vi "z motion pattern_v1.vi"(9 "traj array size":i32, 10 "no of lobes":i8, 11 "Window Array":dbl[](array[numeric])) -> (2 "(cos(n_flr*s/4).^2).*w":dbl[](array[numeric]), 3 "(sin(n_flr*s/4).^2).*w":dbl[](array[numeric]))   [LabVIEW 2010]
uses:
  <vilib>/Analysis/NI_AALBase.lvlib
  <vilib>/Analysis/1siggen.llb/Ramp Pattern by Samples.vi
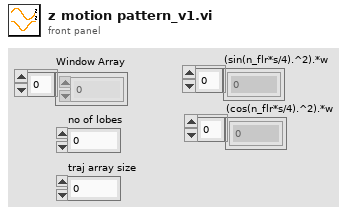
[diagram p1: front panel]
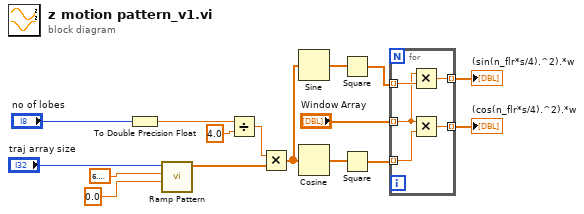
[diagram p0: block diagram]
diagram:
  n1 = To Double Precision Float(number="no of lobes") -> (double precision float=w13:dbl)
  n2 = call-poly <vilib>:"Ramp Pattern.vi"("start"=0.0, "end"=6.283185307179586, "samples"="traj array size") -> ("Ramp Pattern"=w9:dbl[])  [unwired: 7 in, 1 out]
  n3 = Divide(x=w13, y=4.0 ("number")) -> (x/y=w12:dbl)
  n4 = Multiply(x=w12, y=w9) -> (x*y=w6:dbl[])
  n5 = Sine(x=w6) -> (sin(x)=w7:dbl[])
  n6 = Cosine(x=w6) -> (cos(x)=w8:dbl[])
  n7 = Square(x=w7) -> (x^2=w4:dbl[])
  n8 = Square(x=w8) -> (x^2=w3:dbl[])
  n9 = for {
    tunnel: "Window Array" -> [w19] mode=indexing
    tunnel: w4 -> [w21] mode=indexing
    tunnel: w3 -> [w20] mode=indexing
    tunnel: [w18] -> w2 mode=indexing
    tunnel: [w17] -> w1 mode=indexing
    n10 = Multiply(x=w19, y=w21) -> (x*y=w18:dbl)
    n11 = Multiply(x=w19, y=w20) -> (x*y=w17:dbl)
  }
  "(sin(n_flr*s/4).^2).*w" <- w2
  "(cos(n_flr*s/4).^2).*w" <- w1
